vi "ComputeRasterCoordinates_Ant.vi"(6 "antenna angle":dbl=0.2939511935284812 format="%.4f", 8 "TestZT":cluster{"Z mm":dbl, "Horizontal T deg":dbl}={"Z mm"=0.0, "Horizontal T deg"=77.0}, 9 "Center Vector, y and x":dbl[](array[numeric])=[241.68344120684625, 300.8076172317183], 10 "Points per side":dbl=16.0, 11 "Nyquist, mm":dbl=28.0) -> (2 "XY Graph for evaluation":cluster{dbl[], dbl[]}[](graph), 3 "Position Array":T1(array[cluster])=[{"X mm"=90.80761723171833, "Y mm"=31.683441206846254, "Z mm"=0.0, "T deg."=77.0}, {"X mm"=90.95126825422192, "Y mm"=59.68307271127384, "Z mm"=0.0, "T deg."=77.0}, {"X mm"=91.0949192767255, "Y mm"=87.68270421570142, "Z mm"=0.0, "T deg."=77.0}, {"X mm"=91.23857029922911, "Y mm"=115.682335720129, "Z mm"=0.0, "T deg."=77.0}, {"X mm"=91.3822213217327, "Y mm"=143.6819672245566, "Z mm"=0.0, "T deg."=77.0}, {"X mm"=91.52587234423629, "Y mm"=171.68159872898417, "Z mm"=0.0, "T deg."=77.0}, {"X mm"=91.66952336673988, "Y mm"=199.68123023341175, "Z mm"=0.0, "T deg."=77.0}, {"X mm"=91.81317438924347, "Y mm"=227.68086173783934, "Z mm"=0.0, "T deg."=77.0}, {"X mm"=91.95682541174706, "Y mm"=255.68049324226692, "Z mm"=0.0, "T deg."=77.0}, {"X mm"=92.10047643425067, "Y mm"=283.6801247466945, "Z mm"=0.0, "T deg."=77.0}, {"X mm"=92.24412745675426, "Y mm"=311.67975625112206, "Z mm"=0.0, "T deg."=77.0}, {"X mm"=92.38777847925785, "Y mm"=339.67938775554967, "Z mm"=0.0, "T deg."=77.0}, {"X mm"=92.53142950176144, "Y mm"=367.6790192599773, "Z mm"=0.0, "T deg."=77.0}, {"X mm"=92.67508052426503, "Y mm"=395.6786507644049, "Z mm"=0.0, "T deg."=77.0}, {"X mm"=92.81873154676863, "Y mm"=423.6782822688324, "Z mm"=0.0, "T deg."=77.0}, {"X mm"=92.96238256927222, "Y mm"=451.67791377326, "Z mm"=0.0, "T deg."=77.0}, {"X mm"=118.80724873614591, "Y mm"=31.827092229349848, "Z mm"=0.0, "T deg."=77.0}, {"X mm"=118.9508997586495, "Y mm"=59.82672373377743, "Z mm"=0.0, "T deg."=77.0}, {"X mm"=119.09455078115309, "Y mm"=87.82635523820501, "Z mm"=0.0, "T deg."=77.0}, {"X mm"=119.2382018036567, "Y mm"=115.8259867426326, "Z mm"=0.0, "T deg."=77.0}, {"X mm"=119.38185282616028, "Y mm"=143.8256182470602, "Z mm"=0.0, "T deg."=77.0}, {"X mm"=119.52550384866387, "Y mm"=171.82524975148777, "Z mm"=0.0, "T deg."=77.0}, {"X mm"=119.66915487116746, "Y mm"=199.82488125591536, "Z mm"=0.0, "T deg."=77.0}, {"X mm"=119.81280589367105, "Y mm"=227.82451276034294, "Z mm"=0.0, "T deg."=77.0}, {"X mm"=119.95645691617464, "Y mm"=255.82414426477052, "Z mm"=0.0, "T deg."=77.0}, {"X mm"=120.10010793867825, "Y mm"=283.8237757691981, "Z mm"=0.0, "T deg."=77.0}, {"X mm"=120.24375896118184, "Y mm"=311.82340727362566, "Z mm"=0.0, "T deg."=77.0}, {"X mm"=120.38740998368543, "Y mm"=339.8230387780533, "Z mm"=0.0, "T deg."=77.0}, {"X mm"=120.53106100618902, "Y mm"=367.8226702824809, "Z mm"=0.0, "T deg."=77.0}, {"X mm"=120.67471202869261, "Y mm"=395.8223017869085, "Z mm"=0.0, "T deg."=77.0}, {"X mm"=120.81836305119621, "Y mm"=423.821933291336, "Z mm"=0.0, "T deg."=77.0}, {"X mm"=120.9620140736998, "Y mm"=451.8215647957636, "Z mm"=0.0, "T deg."=77.0}, {"X mm"=146.8068802405735, "Y mm"=31.97074325185344, "Z mm"=0.0, "T deg."=77.0}, {"X mm"=146.9505312630771, "Y mm"=59.970374756281025, "Z mm"=0.0, "T deg."=77.0}, {"X mm"=147.09418228558067, "Y mm"=87.9700062607086, "Z mm"=0.0, "T deg."=77.0}, {"X mm"=147.23783330808428, "Y mm"=115.96963776513618, "Z mm"=0.0, "T deg."=77.0}, {"X mm"=147.38148433058785, "Y mm"=143.96926926956377, "Z mm"=0.0, "T deg."=77.0}, {"X mm"=147.52513535309146, "Y mm"=171.96890077399135, "Z mm"=0.0, "T deg."=77.0}, {"X mm"=147.66878637559506, "Y mm"=199.96853227841893, "Z mm"=0.0, "T deg."=77.0}, {"X mm"=147.81243739809864, "Y mm"=227.96816378284652, "Z mm"=0.0, "T deg."=77.0}, {"X mm"=147.95608842060224, "Y mm"=255.9677952872741, "Z mm"=0.0, "T deg."=77.0}, {"X mm"=148.09973944310582, "Y mm"=283.9674267917017, "Z mm"=0.0, "T deg."=77.0}, {"X mm"=148.24339046560942, "Y mm"=311.96705829612927, "Z mm"=0.0, "T deg."=77.0}, {"X mm"=148.38704148811303, "Y mm"=339.9666898005569, "Z mm"=0.0, "T deg."=77.0}, {"X mm"=148.5306925106166, "Y mm"=367.9663213049845, "Z mm"=0.0, "T deg."=77.0}, {"X mm"=148.6743435331202, "Y mm"=395.9659528094121, "Z mm"=0.0, "T deg."=77.0}, {"X mm"=148.81799455562378, "Y mm"=423.9655843138396, "Z mm"=0.0, "T deg."=77.0}, {"X mm"=148.9616455781274, "Y mm"=451.9652158182672, "Z mm"=0.0, "T deg."=77.0}, {"X mm"=174.80651174500107, "Y mm"=32.11439427435703, "Z mm"=0.0, "T deg."=77.0}, {"X mm"=174.95016276750468, "Y mm"=60.114025778784615, "Z mm"=0.0, "T deg."=77.0}, {"X mm"=175.09381379000826, "Y mm"=88.1136572832122, "Z mm"=0.0, "T deg."=77.0}, {"X mm"=175.23746481251186, "Y mm"=116.11328878763979, "Z mm"=0.0, "T deg."=77.0}, {"X mm"=175.38111583501544, "Y mm"=144.11292029206737, "Z mm"=0.0, "T deg."=77.0}, {"X mm"=175.52476685751904, "Y mm"=172.11255179649496, "Z mm"=0.0, "T deg."=77.0}, {"X mm"=175.66841788002264, "Y mm"=200.11218330092254, "Z mm"=0.0, "T deg."=77.0}, {"X mm"=175.81206890252622, "Y mm"=228.11181480535012, "Z mm"=0.0, "T deg."=77.0}, {"X mm"=175.95571992502983, "Y mm"=256.1114463097777, "Z mm"=0.0, "T deg."=77.0}, {"X mm"=176.0993709475334, "Y mm"=284.11107781420526, "Z mm"=0.0, "T deg."=77.0}, {"X mm"=176.243021970037, "Y mm"=312.1107093186328, "Z mm"=0.0, "T deg."=77.0}, {"X mm"=176.3866729925406, "Y mm"=340.1103408230604, "Z mm"=0.0, "T deg."=77.0}, {"X mm"=176.5303240150442, "Y mm"=368.10997232748804, "Z mm"=0.0, "T deg."=77.0}, {"X mm"=176.6739750375478, "Y mm"=396.10960383191565, "Z mm"=0.0, "T deg."=77.0}, {"X mm"=176.81762606005137, "Y mm"=424.10923533634315, "Z mm"=0.0, "T deg."=77.0}, {"X mm"=176.96127708255497, "Y mm"=452.10886684077076, "Z mm"=0.0, "T deg."=77.0}, {"X mm"=202.80614324942866, "Y mm"=32.25804529686062, "Z mm"=0.0, "T deg."=77.0}, {"X mm"=202.94979427193226, "Y mm"=60.257676801288206, "Z mm"=0.0, "T deg."=77.0}, {"X mm"=203.09344529443584, "Y mm"=88.2573083057158, "Z mm"=0.0, "T deg."=77.0}, {"X mm"=203.23709631693944, "Y mm"=116.25693981014338, "Z mm"=0.0, "T deg."=77.0}, {"X mm"=203.38074733944302, "Y mm"=144.25657131457095, "Z mm"=0.0, "T deg."=77.0}, {"X mm"=203.52439836194662, "Y mm"=172.25620281899853, "Z mm"=0.0, "T deg."=77.0}, {"X mm"=203.66804938445023, "Y mm"=200.25583432342611, "Z mm"=0.0, "T deg."=77.0}, {"X mm"=203.8117004069538, "Y mm"=228.2554658278537, "Z mm"=0.0, "T deg."=77.0}, {"X mm"=203.9553514294574, "Y mm"=256.2550973322813, "Z mm"=0.0, "T deg."=77.0}, {"X mm"=204.09900245196098, "Y mm"=284.25472883670886, "Z mm"=0.0, "T deg."=77.0}, {"X mm"=204.2426534744646, "Y mm"=312.2543603411364, "Z mm"=0.0, "T deg."=77.0}, {"X mm"=204.3863044969682, "Y mm"=340.25399184556403, "Z mm"=0.0, "T deg."=77.0}, {"X mm"=204.52995551947177, "Y mm"=368.25362334999164, "Z mm"=0.0, "T deg."=77.0}, {"X mm"=204.67360654197537, "Y mm"=396.25325485441925, "Z mm"=0.0, "T deg."=77.0}, {"X mm"=204.81725756447895, "Y mm"=424.25288635884675, "Z mm"=0.0, "T deg."=77.0}, {"X mm"=204.96090858698255, "Y mm"=452.25251786327436, "Z mm"=0.0, "T deg."=77.0}, {"X mm"=230.80577475385624, "Y mm"=32.40169631936422, "Z mm"=0.0, "T deg."=77.0}, {"X mm"=230.94942577635985, "Y mm"=60.4013278237918, "Z mm"=0.0, "T deg."=77.0}, {"X mm"=231.09307679886342, "Y mm"=88.40095932821939, "Z mm"=0.0, "T deg."=77.0}, {"X mm"=231.23672782136703, "Y mm"=116.40059083264697, "Z mm"=0.0, "T deg."=77.0}, {"X mm"=231.3803788438706, "Y mm"=144.40022233707455, "Z mm"=0.0, "T deg."=77.0}, {"X mm"=231.5240298663742, "Y mm"=172.39985384150214, "Z mm"=0.0, "T deg."=77.0}, {"X mm"=231.6676808888778, "Y mm"=200.39948534592972, "Z mm"=0.0, "T deg."=77.0}, {"X mm"=231.8113319113814, "Y mm"=228.3991168503573, "Z mm"=0.0, "T deg."=77.0}, {"X mm"=231.954982933885, "Y mm"=256.39874835478486, "Z mm"=0.0, "T deg."=77.0}, {"X mm"=232.09863395638857, "Y mm"=284.39837985921247, "Z mm"=0.0, "T deg."=77.0}, {"X mm"=232.24228497889217, "Y mm"=312.39801136364, "Z mm"=0.0, "T deg."=77.0}, {"X mm"=232.38593600139578, "Y mm"=340.39764286806763, "Z mm"=0.0, "T deg."=77.0}, {"X mm"=232.52958702389935, "Y mm"=368.39727437249525, "Z mm"=0.0, "T deg."=77.0}, {"X mm"=232.67323804640296, "Y mm"=396.39690587692286, "Z mm"=0.0, "T deg."=77.0}, {"X mm"=232.81688906890653, "Y mm"=424.39653738135036, "Z mm"=0.0, "T deg."=77.0}, {"X mm"=232.96054009141014, "Y mm"=452.39616888577797, "Z mm"=0.0, "T deg."=77.0}, {"X mm"=258.8054062582838, "Y mm"=32.54534734186781, "Z mm"=0.0, "T deg."=77.0}, {"X mm"=258.94905728078743, "Y mm"=60.54497884629539, "Z mm"=0.0, "T deg."=77.0}, {"X mm"=259.09270830329103, "Y mm"=88.54461035072298, "Z mm"=0.0, "T deg."=77.0}, {"X mm"=259.2363593257946, "Y mm"=116.54424185515056, "Z mm"=0.0, "T deg."=77.0}, {"X mm"=259.3800103482982, "Y mm"=144.54387335957816, "Z mm"=0.0, "T deg."=77.0}, {"X mm"=259.5236613708018, "Y mm"=172.54350486400574, "Z mm"=0.0, "T deg."=77.0}, {"X mm"=259.6673123933054, "Y mm"=200.54313636843332, "Z mm"=0.0, "T deg."=77.0}, {"X mm"=259.810963415809, "Y mm"=228.5427678728609, "Z mm"=0.0, "T deg."=77.0}, {"X mm"=259.95461443831255, "Y mm"=256.54239937728846, "Z mm"=0.0, "T deg."=77.0}, {"X mm"=260.09826546081615, "Y mm"=284.5420308817161, "Z mm"=0.0, "T deg."=77.0}, {"X mm"=260.24191648331976, "Y mm"=312.5416623861436, "Z mm"=0.0, "T deg."=77.0}, {"X mm"=260.38556750582336, "Y mm"=340.54129389057124, "Z mm"=0.0, "T deg."=77.0}, {"X mm"=260.52921852832696, "Y mm"=368.54092539499885, "Z mm"=0.0, "T deg."=77.0}, {"X mm"=260.6728695508305, "Y mm"=396.54055689942646, "Z mm"=0.0, "T deg."=77.0}, {"X mm"=260.8165205733341, "Y mm"=424.54018840385396, "Z mm"=0.0, "T deg."=77.0}, {"X mm"=260.9601715958377, "Y mm"=452.5398199082816, "Z mm"=0.0, "T deg."=77.0}, {"X mm"=286.80503776271144, "Y mm"=32.68899836437141, "Z mm"=0.0, "T deg."=77.0}, {"X mm"=286.94868878521504, "Y mm"=60.68862986879899, "Z mm"=0.0, "T deg."=77.0}, {"X mm"=287.09233980771864, "Y mm"=88.68826137322657, "Z mm"=0.0, "T deg."=77.0}, {"X mm"=287.2359908302222, "Y mm"=116.68789287765415, "Z mm"=0.0, "T deg."=77.0}, {"X mm"=287.3796418527258, "Y mm"=144.68752438208173, "Z mm"=0.0, "T deg."=77.0}, {"X mm"=287.5232928752294, "Y mm"=172.68715588650932, "Z mm"=0.0, "T deg."=77.0}, {"X mm"=287.666943897733, "Y mm"=200.6867873909369, "Z mm"=0.0, "T deg."=77.0}, {"X mm"=287.8105949202366, "Y mm"=228.68641889536448, "Z mm"=0.0, "T deg."=77.0}, {"X mm"=287.95424594274016, "Y mm"=256.68605039979207, "Z mm"=0.0, "T deg."=77.0}, {"X mm"=288.09789696524376, "Y mm"=284.6856819042197, "Z mm"=0.0, "T deg."=77.0}, {"X mm"=288.24154798774737, "Y mm"=312.68531340864723, "Z mm"=0.0, "T deg."=77.0}, {"X mm"=288.385199010251, "Y mm"=340.68494491307484, "Z mm"=0.0, "T deg."=77.0}, {"X mm"=288.5288500327546, "Y mm"=368.68457641750246, "Z mm"=0.0, "T deg."=77.0}, {"X mm"=288.6725010552581, "Y mm"=396.68420792193007, "Z mm"=0.0, "T deg."=77.0}, {"X mm"=288.8161520777617, "Y mm"=424.68383942635757, "Z mm"=0.0, "T deg."=77.0}, {"X mm"=288.95980310026533, "Y mm"=452.6834709307852, "Z mm"=0.0, "T deg."=77.0}, {"X mm"=314.804669267139, "Y mm"=32.832649386875, "Z mm"=0.0, "T deg."=77.0}, {"X mm"=314.9483202896426, "Y mm"=60.83228089130258, "Z mm"=0.0, "T deg."=77.0}, {"X mm"=315.0919713121462, "Y mm"=88.83191239573016, "Z mm"=0.0, "T deg."=77.0}, {"X mm"=315.23562233464975, "Y mm"=116.83154390015774, "Z mm"=0.0, "T deg."=77.0}, {"X mm"=315.37927335715335, "Y mm"=144.83117540458534, "Z mm"=0.0, "T deg."=77.0}, {"X mm"=315.52292437965696, "Y mm"=172.83080690901292, "Z mm"=0.0, "T deg."=77.0}, {"X mm"=315.66657540216056, "Y mm"=200.8304384134405, "Z mm"=0.0, "T deg."=77.0}, {"X mm"=315.81022642466417, "Y mm"=228.8300699178681, "Z mm"=0.0, "T deg."=77.0}, {"X mm"=315.9538774471677, "Y mm"=256.82970142229567, "Z mm"=0.0, "T deg."=77.0}, {"X mm"=316.0975284696713, "Y mm"=284.8293329267232, "Z mm"=0.0, "T deg."=77.0}, {"X mm"=316.2411794921749, "Y mm"=312.8289644311508, "Z mm"=0.0, "T deg."=77.0}, {"X mm"=316.3848305146785, "Y mm"=340.8285959355784, "Z mm"=0.0, "T deg."=77.0}, {"X mm"=316.52848153718213, "Y mm"=368.828227440006, "Z mm"=0.0, "T deg."=77.0}, {"X mm"=316.6721325596857, "Y mm"=396.8278589444336, "Z mm"=0.0, "T deg."=77.0}, {"X mm"=316.8157835821893, "Y mm"=424.8274904488611, "Z mm"=0.0, "T deg."=77.0}, {"X mm"=316.9594346046929, "Y mm"=452.8271219532887, "Z mm"=0.0, "T deg."=77.0}, {"X mm"=342.80430077156655, "Y mm"=32.97630040937859, "Z mm"=0.0, "T deg."=77.0}, {"X mm"=342.94795179407015, "Y mm"=60.97593191380617, "Z mm"=0.0, "T deg."=77.0}, {"X mm"=343.09160281657375, "Y mm"=88.97556341823376, "Z mm"=0.0, "T deg."=77.0}, {"X mm"=343.2352538390773, "Y mm"=116.97519492266134, "Z mm"=0.0, "T deg."=77.0}, {"X mm"=343.3789048615809, "Y mm"=144.9748264270889, "Z mm"=0.0, "T deg."=77.0}, {"X mm"=343.5225558840845, "Y mm"=172.9744579315165, "Z mm"=0.0, "T deg."=77.0}, {"X mm"=343.6662069065881, "Y mm"=200.97408943594408, "Z mm"=0.0, "T deg."=77.0}, {"X mm"=343.8098579290917, "Y mm"=228.97372094037166, "Z mm"=0.0, "T deg."=77.0}, {"X mm"=343.95350895159527, "Y mm"=256.9733524447993, "Z mm"=0.0, "T deg."=77.0}, {"X mm"=344.0971599740989, "Y mm"=284.97298394922683, "Z mm"=0.0, "T deg."=77.0}, {"X mm"=344.2408109966025, "Y mm"=312.9726154536544, "Z mm"=0.0, "T deg."=77.0}, {"X mm"=344.3844620191061, "Y mm"=340.972246958082, "Z mm"=0.0, "T deg."=77.0}, {"X mm"=344.5281130416097, "Y mm"=368.9718784625096, "Z mm"=0.0, "T deg."=77.0}, {"X mm"=344.67176406411323, "Y mm"=396.9715099669372, "Z mm"=0.0, "T deg."=77.0}, {"X mm"=344.81541508661684, "Y mm"=424.9711414713647, "Z mm"=0.0, "T deg."=77.0}, {"X mm"=344.95906610912044, "Y mm"=452.97077297579233, "Z mm"=0.0, "T deg."=77.0}, {"X mm"=370.80393227599416, "Y mm"=33.119951431882185, "Z mm"=0.0, "T deg."=77.0}, {"X mm"=370.94758329849776, "Y mm"=61.11958293630977, "Z mm"=0.0, "T deg."=77.0}, {"X mm"=371.09123432100137, "Y mm"=89.11921444073735, "Z mm"=0.0, "T deg."=77.0}, {"X mm"=371.2348853435049, "Y mm"=117.11884594516494, "Z mm"=0.0, "T deg."=77.0}, {"X mm"=371.3785363660085, "Y mm"=145.11847744959252, "Z mm"=0.0, "T deg."=77.0}, {"X mm"=371.5221873885121, "Y mm"=173.1181089540201, "Z mm"=0.0, "T deg."=77.0}, {"X mm"=371.6658384110157, "Y mm"=201.11774045844768, "Z mm"=0.0, "T deg."=77.0}, {"X mm"=371.80948943351933, "Y mm"=229.11737196287527, "Z mm"=0.0, "T deg."=77.0}, {"X mm"=371.9531404560229, "Y mm"=257.1170034673028, "Z mm"=0.0, "T deg."=77.0}, {"X mm"=372.0967914785265, "Y mm"=285.11663497173043, "Z mm"=0.0, "T deg."=77.0}, {"X mm"=372.2404425010301, "Y mm"=313.116266476158, "Z mm"=0.0, "T deg."=77.0}, {"X mm"=372.3840935235337, "Y mm"=341.1158979805856, "Z mm"=0.0, "T deg."=77.0}, {"X mm"=372.5277445460373, "Y mm"=369.1155294850132, "Z mm"=0.0, "T deg."=77.0}, {"X mm"=372.67139556854085, "Y mm"=397.1151609894408, "Z mm"=0.0, "T deg."=77.0}, {"X mm"=372.81504659104445, "Y mm"=425.1147924938683, "Z mm"=0.0, "T deg."=77.0}, {"X mm"=372.95869761354805, "Y mm"=453.11442399829593, "Z mm"=0.0, "T deg."=77.0}, {"X mm"=398.8035637804217, "Y mm"=33.263602454385776, "Z mm"=0.0, "T deg."=77.0}, {"X mm"=398.9472148029253, "Y mm"=61.26323395881336, "Z mm"=0.0, "T deg."=77.0}, {"X mm"=399.0908658254289, "Y mm"=89.26286546324094, "Z mm"=0.0, "T deg."=77.0}, {"X mm"=399.23451684793247, "Y mm"=117.26249696766853, "Z mm"=0.0, "T deg."=77.0}, {"X mm"=399.3781678704361, "Y mm"=145.26212847209612, "Z mm"=0.0, "T deg."=77.0}, {"X mm"=399.5218188929397, "Y mm"=173.2617599765237, "Z mm"=0.0, "T deg."=77.0}, {"X mm"=399.6654699154433, "Y mm"=201.2613914809513, "Z mm"=0.0, "T deg."=77.0}, {"X mm"=399.8091209379469, "Y mm"=229.26102298537887, "Z mm"=0.0, "T deg."=77.0}, {"X mm"=399.95277196045043, "Y mm"=257.2606544898064, "Z mm"=0.0, "T deg."=77.0}, {"X mm"=400.09642298295404, "Y mm"=285.26028599423404, "Z mm"=0.0, "T deg."=77.0}, {"X mm"=400.24007400545764, "Y mm"=313.2599174986616, "Z mm"=0.0, "T deg."=77.0}, {"X mm"=400.38372502796125, "Y mm"=341.2595490030892, "Z mm"=0.0, "T deg."=77.0}, {"X mm"=400.52737605046485, "Y mm"=369.2591805075168, "Z mm"=0.0, "T deg."=77.0}, {"X mm"=400.6710270729684, "Y mm"=397.2588120119444, "Z mm"=0.0, "T deg."=77.0}, {"X mm"=400.814678095472, "Y mm"=425.2584435163719, "Z mm"=0.0, "T deg."=77.0}, {"X mm"=400.9583291179756, "Y mm"=453.25807502079954, "Z mm"=0.0, "T deg."=77.0}, {"X mm"=426.8031952848493, "Y mm"=33.407253476889366, "Z mm"=0.0, "T deg."=77.0}, {"X mm"=426.9468463073529, "Y mm"=61.40688498131695, "Z mm"=0.0, "T deg."=77.0}, {"X mm"=427.09049732985653, "Y mm"=89.40651648574453, "Z mm"=0.0, "T deg."=77.0}, {"X mm"=427.2341483523601, "Y mm"=117.40614799017212, "Z mm"=0.0, "T deg."=77.0}, {"X mm"=427.3777993748637, "Y mm"=145.4057794945997, "Z mm"=0.0, "T deg."=77.0}, {"X mm"=427.5214503973673, "Y mm"=173.40541099902728, "Z mm"=0.0, "T deg."=77.0}, {"X mm"=427.6651014198709, "Y mm"=201.40504250345487, "Z mm"=0.0, "T deg."=77.0}, {"X mm"=427.8087524423745, "Y mm"=229.40467400788245, "Z mm"=0.0, "T deg."=77.0}, {"X mm"=427.95240346487805, "Y mm"=257.40430551231003, "Z mm"=0.0, "T deg."=77.0}, {"X mm"=428.09605448738165, "Y mm"=285.40393701673764, "Z mm"=0.0, "T deg."=77.0}, {"X mm"=428.23970550988525, "Y mm"=313.4035685211652, "Z mm"=0.0, "T deg."=77.0}, {"X mm"=428.38335653238886, "Y mm"=341.4032000255928, "Z mm"=0.0, "T deg."=77.0}, {"X mm"=428.52700755489246, "Y mm"=369.4028315300204, "Z mm"=0.0, "T deg."=77.0}, {"X mm"=428.670658577396, "Y mm"=397.40246303444803, "Z mm"=0.0, "T deg."=77.0}, {"X mm"=428.8143095998996, "Y mm"=425.40209453887553, "Z mm"=0.0, "T deg."=77.0}, {"X mm"=428.9579606224032, "Y mm"=453.40172604330314, "Z mm"=0.0, "T deg."=77.0}, {"X mm"=454.80282678927693, "Y mm"=33.55090449939296, "Z mm"=0.0, "T deg."=77.0}, {"X mm"=454.94647781178054, "Y mm"=61.55053600382055, "Z mm"=0.0, "T deg."=77.0}, {"X mm"=455.09012883428414, "Y mm"=89.55016750824812, "Z mm"=0.0, "T deg."=77.0}, {"X mm"=455.2337798567877, "Y mm"=117.5497990126757, "Z mm"=0.0, "T deg."=77.0}, {"X mm"=455.3774308792913, "Y mm"=145.5494305171033, "Z mm"=0.0, "T deg."=77.0}, {"X mm"=455.5210819017949, "Y mm"=173.5490620215309, "Z mm"=0.0, "T deg."=77.0}, {"X mm"=455.6647329242985, "Y mm"=201.54869352595847, "Z mm"=0.0, "T deg."=77.0}, {"X mm"=455.8083839468021, "Y mm"=229.54832503038605, "Z mm"=0.0, "T deg."=77.0}, {"X mm"=455.95203496930566, "Y mm"=257.54795653481364, "Z mm"=0.0, "T deg."=77.0}, {"X mm"=456.09568599180926, "Y mm"=285.5475880392412, "Z mm"=0.0, "T deg."=77.0}, {"X mm"=456.23933701431287, "Y mm"=313.54721954366875, "Z mm"=0.0, "T deg."=77.0}, {"X mm"=456.38298803681647, "Y mm"=341.54685104809636, "Z mm"=0.0, "T deg."=77.0}, {"X mm"=456.5266390593201, "Y mm"=369.54648255252397, "Z mm"=0.0, "T deg."=77.0}, {"X mm"=456.6702900818236, "Y mm"=397.5461140569516, "Z mm"=0.0, "T deg."=77.0}, {"X mm"=456.8139411043272, "Y mm"=425.5457455613791, "Z mm"=0.0, "T deg."=77.0}, {"X mm"=456.95759212683083, "Y mm"=453.5453770658067, "Z mm"=0.0, "T deg."=77.0}, {"X mm"=482.8024582937045, "Y mm"=33.694555521896554, "Z mm"=0.0, "T deg."=77.0}, {"X mm"=482.9461093162081, "Y mm"=61.69418702632414, "Z mm"=0.0, "T deg."=77.0}, {"X mm"=483.0897603387117, "Y mm"=89.69381853075173, "Z mm"=0.0, "T deg."=77.0}, {"X mm"=483.23341136121525, "Y mm"=117.69345003517931, "Z mm"=0.0, "T deg."=77.0}, {"X mm"=483.37706238371885, "Y mm"=145.69308153960688, "Z mm"=0.0, "T deg."=77.0}, {"X mm"=483.52071340622246, "Y mm"=173.69271304403446, "Z mm"=0.0, "T deg."=77.0}, {"X mm"=483.66436442872606, "Y mm"=201.69234454846205, "Z mm"=0.0, "T deg."=77.0}, {"X mm"=483.80801545122966, "Y mm"=229.69197605288963, "Z mm"=0.0, "T deg."=77.0}, {"X mm"=483.9516664737332, "Y mm"=257.69160755731724, "Z mm"=0.0, "T deg."=77.0}, {"X mm"=484.0953174962368, "Y mm"=285.6912390617448, "Z mm"=0.0, "T deg."=77.0}, {"X mm"=484.2389685187404, "Y mm"=313.69087056617235, "Z mm"=0.0, "T deg."=77.0}, {"X mm"=484.382619541244, "Y mm"=341.69050207059996, "Z mm"=0.0, "T deg."=77.0}, {"X mm"=484.52627056374763, "Y mm"=369.6901335750276, "Z mm"=0.0, "T deg."=77.0}, {"X mm"=484.6699215862512, "Y mm"=397.6897650794552, "Z mm"=0.0, "T deg."=77.0}, {"X mm"=484.8135726087548, "Y mm"=425.6893965838827, "Z mm"=0.0, "T deg."=77.0}, {"X mm"=484.9572236312584, "Y mm"=453.6890280883103, "Z mm"=0.0, "T deg."=77.0}, {"X mm"=510.80208979813204, "Y mm"=33.83820654440015, "Z mm"=0.0, "T deg."=77.0}, {"X mm"=510.94574082063565, "Y mm"=61.837838048827734, "Z mm"=0.0, "T deg."=77.0}, {"X mm"=511.08939184313925, "Y mm"=89.83746955325532, "Z mm"=0.0, "T deg."=77.0}, {"X mm"=511.2330428656428, "Y mm"=117.8371010576829, "Z mm"=0.0, "T deg."=77.0}, {"X mm"=511.3766938881464, "Y mm"=145.83673256211048, "Z mm"=0.0, "T deg."=77.0}, {"X mm"=511.52034491065, "Y mm"=173.83636406653807, "Z mm"=0.0, "T deg."=77.0}, {"X mm"=511.6639959331536, "Y mm"=201.83599557096565, "Z mm"=0.0, "T deg."=77.0}, {"X mm"=511.8076469556572, "Y mm"=229.83562707539323, "Z mm"=0.0, "T deg."=77.0}, {"X mm"=511.95129797816077, "Y mm"=257.8352585798208, "Z mm"=0.0, "T deg."=77.0}, {"X mm"=512.0949490006644, "Y mm"=285.8348900842484, "Z mm"=0.0, "T deg."=77.0}, {"X mm"=512.2386000231679, "Y mm"=313.83452158867595, "Z mm"=0.0, "T deg."=77.0}, {"X mm"=512.3822510456715, "Y mm"=341.83415309310357, "Z mm"=0.0, "T deg."=77.0}, {"X mm"=512.5259020681751, "Y mm"=369.8337845975312, "Z mm"=0.0, "T deg."=77.0}, {"X mm"=512.6695530906787, "Y mm"=397.8334161019588, "Z mm"=0.0, "T deg."=77.0}, {"X mm"=512.8132041131823, "Y mm"=425.8330476063863, "Z mm"=0.0, "T deg."=77.0}, {"X mm"=512.9568551356859, "Y mm"=453.8326791108139, "Z mm"=0.0, "T deg."=77.0}])   [LabVIEW 2018]
doc: "This version is aligned to the Antenna axes.\nIf the antenna is rotated slightly, ~ 1 degrees, this raster will have that rotation."
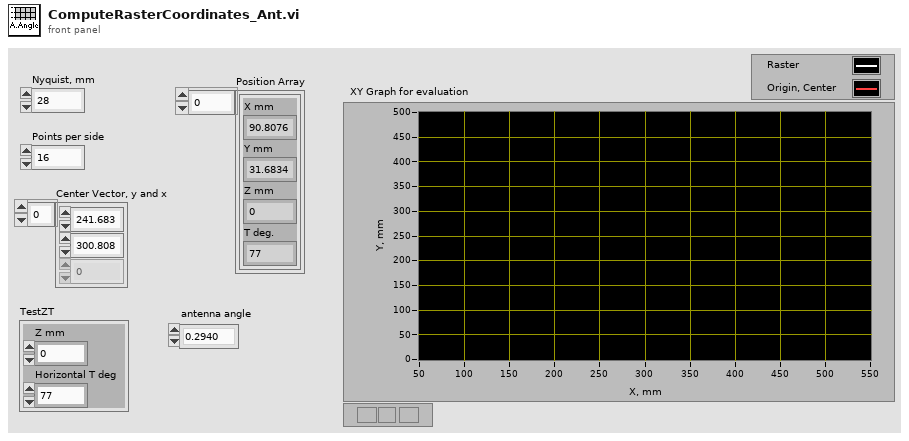
[diagram p1: front panel]
types:
  T1 = cluster{"X mm":dbl, "Y mm":dbl, "Z mm":dbl, "T deg.":dbl}[]
  T2 = cluster{"X mm":dbl, "Y mm":dbl, "Z mm":dbl, "T deg.":dbl}
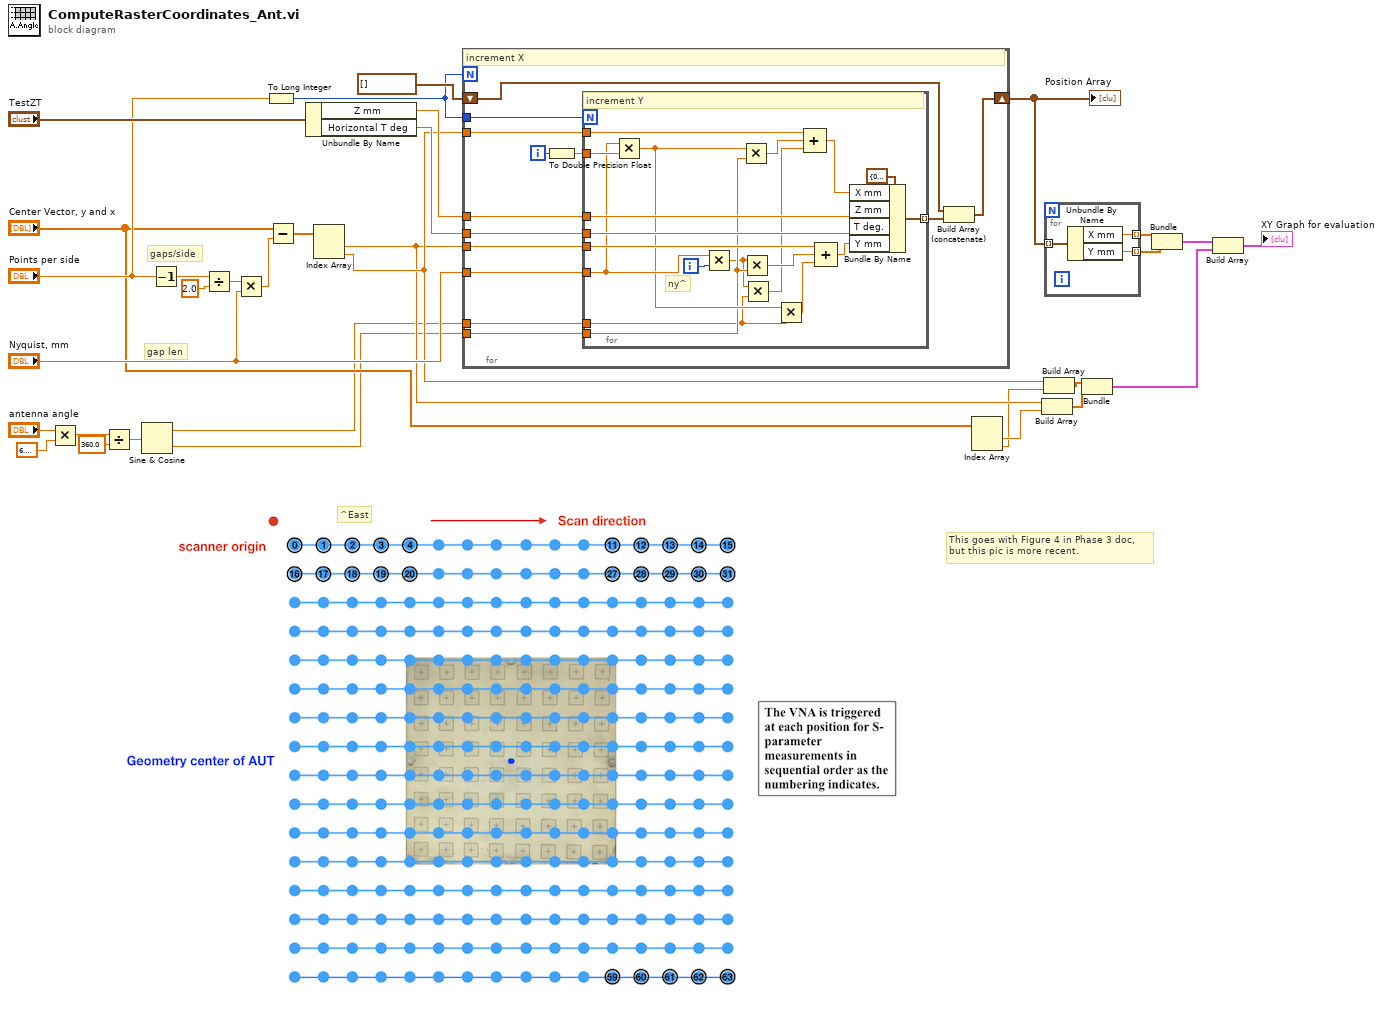
[diagram p0: block diagram]
diagram:
  # "^East"
  # "gap len"
  # "gaps/side"
  # "This goes with Figure 4 in Phase 3 doc,\nbut this pic is more recent."
  n1 = Multiply(x="antenna angle", y=6.283185307179586) -> (x*y=w5:dbl)
  n2 = Divide(x=w5, y=360.0) -> (x/y=w3:dbl)
  n3 = Sine & Cosine(0:w3) -> (1:w1:dbl, 2:w2:dbl)
  n4 = Decrement(x="Points per side") -> (x-1=w9:dbl)
  n5 = Divide(x=w9, y=2.0) -> (x/y=w27:dbl)
  n6 = Multiply(x=w27, y="Nyquist, mm") -> (x*y=w31:dbl)
  n7 = To Long Integer(number="Points per side") -> (32bit integer=w22:i32)
  n8 = Subtract(x="Center Vector, y and x", y=w31) -> (x-y=w26:dbl[])
  n9 = Unbundle By Name("TestZT") -> ("Z mm"=w28:dbl, "Horizontal T deg"=w25:dbl)
  n10 = Index Array(array=w26) -> (element #1=w16:dbl, element #2=w17:dbl)  [unwired: 2 in]
  n11 = for {
    N: w22 -> [_]
    tunnel: "Nyquist, mm" -> [w42]
    tunnel: w22 -> [w45]
    shift-right: [w44] -> w21
    shift-left: T1 [] -> [w33]
    tunnel: w28 -> [w39]
    tunnel: w25 -> [w38]
    tunnel: w16 -> [w41]
    tunnel: w17 -> [w37]
    tunnel: w2 -> [w40]
    tunnel: w1 -> [w35]
    i -> [w36]
    # "increment X"
    n12 = To Double Precision Float(number=w36) -> (double precision float=w34:dbl)
    n13 = for {
      N: w45 -> [_]
      tunnel: w41 -> [w64]
      tunnel: w42 -> [w55]
      tunnel: [w62] -> w43 mode=indexing
      tunnel: w40 -> [w50]
      tunnel: w39 -> [w59]
      tunnel: w38 -> [w58]
      tunnel: w37 -> [w57]
      tunnel: w34 -> [w56]
      tunnel: w35 -> [w47]
      i -> [w63]
      # "ny^"
      # "increment Y"
      n14 = Multiply(x=w55, y=w56) -> (x*y=w51:dbl)
      n15 = Multiply(x=w55, y=w63) -> (x*y=w48:dbl)
      n16 = Multiply(x=w51, y=w50) -> (x*y=w49:dbl)
      n17 = Multiply(x=w48, y=w50) -> (x*y=w52:dbl)
      n18 = Multiply(x=w48, y=w47) -> (x*y=w46:dbl)
      n19 = Multiply(x=w51, y=w47) -> (x*y=w53:dbl)
      n20 = Compound Arithmetic op=ADD(w57, w49, w46) -> (w54:dbl)
      n21 = Compound Arithmetic op=ADD(w64, w52, w53) -> (w61:dbl)
      n22 = Bundle By Name(cluster=T2 {"X mm"=0.0, "Y mm"=0.0, "Z mm"=0.0, "T deg."=0.0} ("Position 15"), "X mm"=w54, "Z mm"=w59, "T deg."=w58, "Y mm"=w61) -> (w62:T2)
    }
    n23 = Build Array (concatenate)(w33, w43) -> (w44:T1)
  }
  "Position Array" <- w21
  n24 = Index Array(array="Center Vector, y and x") -> (element #1=w11:dbl, element #2=w10:dbl)  [unwired: 2 in]
  n25 = Build Array(w16, w11) -> (w14:dbl[])
  n26 = Build Array(w17, w10) -> (w15:dbl[])
  n27 = for {
    tunnel: w21 -> [w67] mode=indexing
    tunnel: [w66] -> w20 mode=indexing
    tunnel: [w65] -> w19 mode=indexing
    n28 = Unbundle By Name(w67) -> ("X mm"=w66:dbl, "Y mm"=w65:dbl)
  }
  n29 = Bundle(w15, w14) -> (w12:cluster{dbl[], dbl[]})  [unwired: 1 in]
  n30 = Bundle(w20, w19) -> (w18:cluster{dbl[], dbl[]})  [unwired: 1 in]
  n31 = Build Array(w18, w12) -> (→"XY Graph for evaluation":cluster{dbl[], dbl[]}[])
